vi "Certify_Change.vi"(8 "error in (no error)":errorcluster, 9 "Variable Name":string, 10 "New Value":variant, 11 "Default Value":variant) -> (0 "error out":errorcluster, 3 "Value Out":variant)   [LabVIEW 2013]
doc: "Asks the user if they are certain they want to change a variable from an old value to a given new value. WIRE THE OUTPUT OF THIS VI TO Connection>Database>Database Variant to Value.vi. If the given values are the same or the vi is fed an error, this vi will output whatever is wired to Default Value."
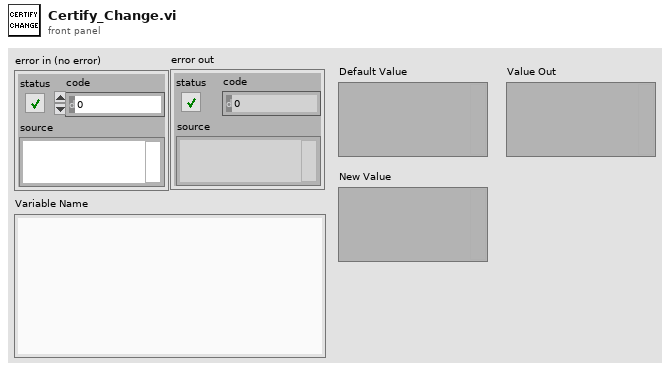
[diagram p1: front panel]
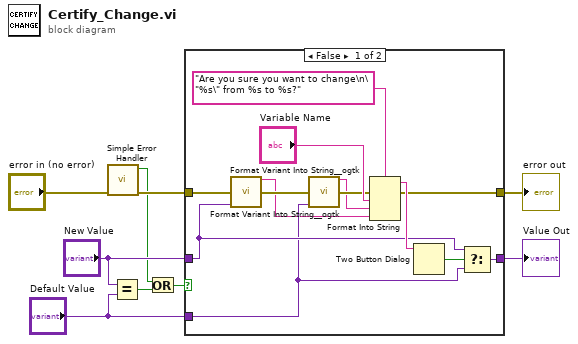
[diagram p0: block diagram]
diagram:
  n1 = call <vilib>:"Simple Error Handler.vi"("error in (no error)"="error in (no error)") -> ("error?"=w1:bool, "error out"=w4:errorcluster)  [unwired: 4 in, 3 out]
  n2 = Equal?(x="New Value", y="Default Value") -> (x = y?=w2:bool)
  n3 = Or(x=w1, y=w2) -> (x .or. y?=w3:bool)
  n4 = case shown="False" w3 {
    tunnel: "New Value" -> [w15 _]
    tunnel: "Default Value" -> [w14 w23]
    tunnel: w4 -> [w19 w24]
    tunnel: [w13 w23] -> w6
    tunnel: [w12 w24] -> w5
    frame False {
      n5 = call <userlib>:"Format Variant Into String__ogtk.vi"("error in (no error)"=w19, "Variant"=w15) -> ("Output String"=w10:string, "error out"=w18:errorcluster)  [unwired: 12 in]
      n6 = call <userlib>:"Format Variant Into String__ogtk.vi"("error in (no error)"=w18, "Variant"=w14) -> ("Output String"=w11:string, "error out"=w17:errorcluster)  [unwired: 12 in]
      n7 = Format Into String(format string="Are you sure you want to change\n\"%s\" from %s to %s?", error in=w17, "Variable Name", w11, w10) -> (resulting string=w20:string, error out=w12:errorcluster)  [unwired: 1 in]
      n8 = Two Button Dialog(message=w20) -> (T button?=w16:bool)  [unwired: 2 in]
      n9 = Select(t=w15, s=w16, f=w14) -> (s? t:f=w13:variant)
    }
    frame True {
    }
  }
  "error out" <- w5
  "Value Out" <- w6
